vi "Delay DeBounce.vi"(7 "Enable":bool=TRUE, 8 "error in":errorcluster, 10 "preset time (ms)":u32=20, 11 "Input":bool) -> (0 "error out":errorcluster, 3 "Output":bool)   [LabVIEW 2012]
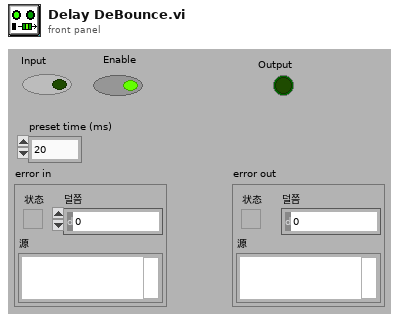
[diagram p1: front panel]
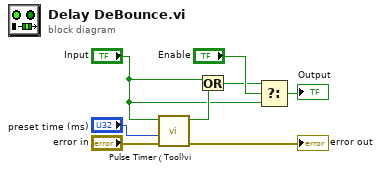
[diagram p0: block diagram]
diagram:
  n1 = call "Pulse Timer（Tool)vi.vi"("error in"="error in", "preset time (ms)"="preset time (ms)", "input"="Input") -> ("error out"=→"error out":errorcluster, "output"=w5:bool)  [unwired: 6 in, 1 out]
  n2 = Or(x="Input", y=w5) -> (x .or. y?=w4:bool)
  n3 = Select(t=w4, s="Enable", f="Input") -> (s? t:f=→"Output":bool)
